vi "Publish Data.vi"() -> (0 "error out":errorcluster, 4 "log":string)   [LabVIEW 2024]
uses:
  <vilib>/Plug-In SDKs/Clients/Data Store V1/Data Store Client.lvlibp/API/Data Store V1/Test Result.ctl
  <vilib>/Plug-In SDKs/Clients/Metadata/Outcome.ctl
  <vilib>/Plug-In SDKs/Clients/Metadata/Extension.ctl
  Test Result Info.ctl
  <vilib>/Plug-In SDKs/Clients/Metadata/Step.ctl
  <vilib>/numeric/Random Number (Range) DBL.vi
  <vilib>/Plug-In SDKs/Clients/Data Store V1/Data Store Client.lvlibp/API/Data Store V1/Publish Measurement (DBL).vi
  <vilib>/Plug-In SDKs/Clients/Data Store V1/Data Store Client.lvlibp/API/Data Store V1/Publish Condition (Double).vi
  <vilib>/Plug-In SDKs/Clients/Data Store V1/Data Store Client.lvlibp
  <vilib>/Plug-In SDKs/Clients/Metadata/NI Metadata Types.lvlib
panel:
  # "Publish Data\n\nCreates and publishes data and metadata items that can be queried using the other VIs in this example."
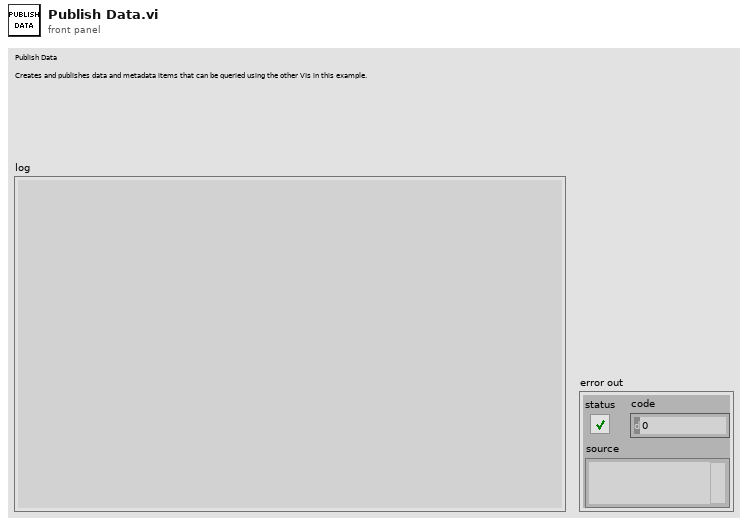
[diagram p1: front panel]
types:
  T1 = typedef "Data Store Client.lvlibp/Test Result.ctl" = cluster{"test result name":string, "start date time":timestamp, "end date time":timestamp, "outcome":T2, "test result id":string, "uut instance id":string, "operator id":string, "test station id":string, "test description id":string, "software item ids":string[], "hardware item ids":string[], "test adapter ids":string[], "link":string, "extensions":T3[], "schema id":string}
  T2 = typedef "NI Metadata Types.lvlib/Outcome.ctl" = enum32{"Unspecified", "Passed", "Failed", "Indeterminate"}
  T3 = typedef "NI Metadata Types.lvlib/Extension.ctl" = cluster{"name":string, "value":string}
  T4 = typedef "Test Result Info.ctl" = cluster{"Name":string, "Measurements":cluster{"Name":string, "Min_Value":dbl, "Max_Value":dbl, "Units":string}[], "Conditions":cluster{"Name":string, "Min_Value":dbl, "Max_Value":dbl, "Units":string}[]}[]
  T5 = typedef "NI Metadata Types.lvlib/Step.ctl" = cluster{"step name":string, "step type":string, "start date time":timestamp, "end date time":timestamp, "notes":string, "step id":string, "parent step id":string, "test result id":string, "test id":string, "link":string, "extensions":T3[], "schema id":string}
  T6 = cluster{"Name":string, "Min_Value":dbl, "Max_Value":dbl, "Units":string}[]
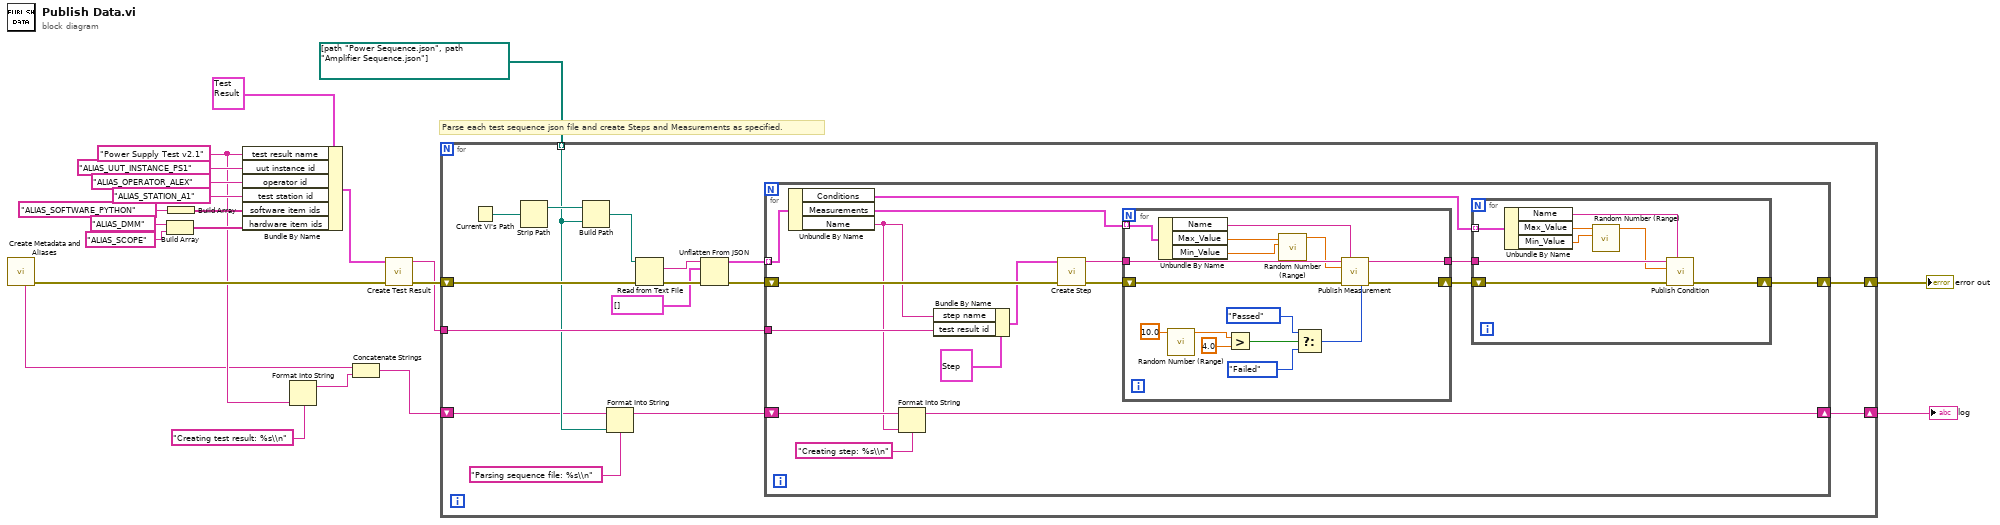
[diagram p0: block diagram]
diagram:
  w5 = "Power Supply Test v2.1" ("test result name")
  # "Parse each test sequence json file and create Steps and Measurements as specified."
  n1 = call "Create Metadata and Aliases.vi"() -> ("error out"=w11:errorcluster, "log"=w4:string)  [unwired: 10 in]
  n2 = Build Array("ALIAS_DMM" ("test station id"), "ALIAS_SCOPE" ("element")) -> (w14:string[])
  n3 = Build Array("ALIAS_SOFTWARE_PYTHON" ("test station id")) -> (w16:string[])
  n4 = Bundle By Name(cluster=T1 {"test result name"="", "start date time"=timestamp(0 s since 1904-01-01), "end date time"=timestamp(0 s since 1904-01-01), "outcome"=enum."Unspecified", "test result id"="", "uut instance id"="", "operator id"="", "test station id"="", "test description id"="", "software item ids"=[], "hardware item ids"=[], "test adapter ids"=[], "link"="", "extensions"=[], "schema id"=""} ("test result"), "test result name"=w5, "uut instance id"="ALIAS_UUT_INSTANCE_PS1", "operator id"="ALIAS_OPERATOR_ALEX", "test station id"="ALIAS_STATION_A1", "software item ids"=w16, "hardware item ids"=w14) -> (w12:T1)
  n5 = Format Into String(format string="Creating test result: %s\\n", w5) -> (resulting string=w3:string)  [unwired: 2 in, 1 out]
  n6 = Concatenate Strings(w4, w3) -> (w2:string)
  n7 = call <vilib>:"Create Test Result.vi"("error in"=w11, "test result"=w12) -> ("error out"=w10:errorcluster, "test result id"=w8:string)  [unwired: 8 in]
  n8 = for {
    tunnel: path[] [path "Power Sequence.json", path "Amplifier Sequence.json"] -> [w25] mode=indexing
    tunnel: w8 -> [w29]
    shift-right: [w28] -> w7
    shift-left: w10 -> [w37]
    shift-right: [w22] -> w1
    shift-left: w2 -> [w24]
    n9 = Current VI's Path() -> (path=w36:path)
    n10 = Strip Path(path=w36) -> (stripped path=w35:path)  [unwired: 1 out]
    n11 = Build Path(base path=w35, name or relative path=w25) -> (appended path=w34:path)
    n12 = Format Into String(format string="Parsing sequence file: %s\\n", initial string=w24, w25) -> (resulting string=w23:string)  [unwired: 1 in, 1 out]
    n13 = Read from Text File(file (use dialog)=w34, error in=w37) -> (text=w32:string, error out=w33:errorcluster)  [unwired: 2 in, 2 out]
    n14 = Unflatten From JSON(JSON string=w32, type and defaults=T4 [] ("Steps"), error in (no error)=w33) -> (value=w30:T4, error out=w31:errorcluster)  [unwired: 4 in]
    n15 = for {
      shift-right: [w43] -> w28
      shift-left: w31 -> [w52]
      tunnel: w30 -> [w53] mode=indexing
      tunnel: w29 -> [w50]
      shift-right: [w38] -> w22
      shift-left: w23 -> [w41]
      n16 = Unbundle By Name(w53) -> ("Conditions"=w42:T6, "Measurements"=w48:T6, "Name"=w39:string)
      n17 = Format Into String(format string="Creating step: %s\\n", initial string=w41, w39) -> (resulting string=w38:string)  [unwired: 1 in, 1 out]
      n18 = Bundle By Name(cluster=T5 {"step name"="", "step type"="", "start date time"=timestamp(0 s since 1904-01-01), "end date time"=timestamp(0 s since 1904-01-01), "notes"="", "step id"="", "parent step id"="", "test result id"="", "test id"="", "link"="", "extensions"=[], "schema id"=""} ("step"), "step name"=w39, "test result id"=w50) -> (w49:T5)
      n19 = call <vilib>:"Create Step.vi"("error in"=w52, "step"=w49) -> ("error out"=w45:errorcluster, "step id"=w47:string)  [unwired: 8 in]
      n20 = for {
        tunnel: w48 -> [w77] mode=indexing
        tunnel: w47 -> [w75]
        tunnel: [w70] -> w46
        shift-right: [w71] -> w44
        shift-left: w45 -> [w69]
        n21 = Unbundle By Name(w77) -> ("Name"=w76:string, "Max_Value"=w74:dbl, "Min_Value"=w73:dbl)
        n22 = call-poly <vilib>:"Random Number (Range).vi"("upper bound (100)"=10.0) -> ("number"=w67:dbl)  [unwired: 10 in]
        n23 = Greater?(x=w67, y=4.0) -> (0:w65:bool)
        n24 = call-poly <vilib>:"Random Number (Range).vi"("lower bound (0)"=w73, "upper bound (100)"=w74) -> ("number"=w72:dbl)  [unwired: 9 in]
        n25 = Select(t=Outcome."Passed" ("outcome"), s=w65, f=Outcome."Failed" ("outcome")) -> (s? t:f=w62:T2)
        n26 = call-poly <vilib>:"Publish Measurement.vi"("step id"=w75, "name"=w76, "outcome"=w62, "value"=w72, "error in"=w69) -> ("step id out"=w70:string, "error out"=w71:errorcluster)  [unwired: 8 in, 1 out]
      }
      n27 = for {
        tunnel: w42 -> [w61] mode=indexing
        tunnel: w46 -> [w59]
        shift-right: [w54] -> w43
        shift-left: w44 -> [w58]
        n28 = Unbundle By Name(w61) -> ("Name"=w60:string, "Max_Value"=w57:dbl, "Min_Value"=w56:dbl)
        n29 = call-poly <vilib>:"Random Number (Range).vi"("lower bound (0)"=w56, "upper bound (100)"=w57) -> ("number"=w55:dbl)  [unwired: 9 in]
        n30 = call-poly <vilib>:"Publish Condition.vi"("name"=w60, "error in"=w58, "value"=w55, "step id"=w59) -> ("error out"=w54:errorcluster)  [unwired: 5 in, 2 out]
      }
    }
  }
  "error out" <- w7
  "log" <- w1
